vi "Configure Channel.vi"(4 "Vertical Offset (0.0 V)":dbl format="%.3p", 5 "Vertical Coupling (DC)":i32(slide)=1, 6 "Vertical Range (10.0 V)":dbl=10.0 format="%.2p", 7 "Channel Enabled (True)":bool=TRUE, 8 "error in (no error)":errorcluster {"code" format="%.0x"}, 9 "Probe Attenuation (1.0)":dbl=1.0 format="%.2f", 10 "Channel Name (\"CH1\")":string(combo)="CH1", 11 "VISA Resource Name":refnum<visa-resource-name>) -> (0 "error out":errorcluster {"code" format="%.0x"}, 3 "VISA Resource Name Out":refnum<visa-resource-name>)   [LabVIEW 2010, in "Tektronix TDS 3000 Series.lvlib"]
doc: "This VI configures the common properties of the oscilloscope's channel subsystem for a particular channel. These properties are the vertical range, vertical offset, coupling, probe attenuation, and channel enabled."
uses:
  <instrlib>/Tektronix TDS 3000 Series/Tektronix TDS 3000 Series.lvlib
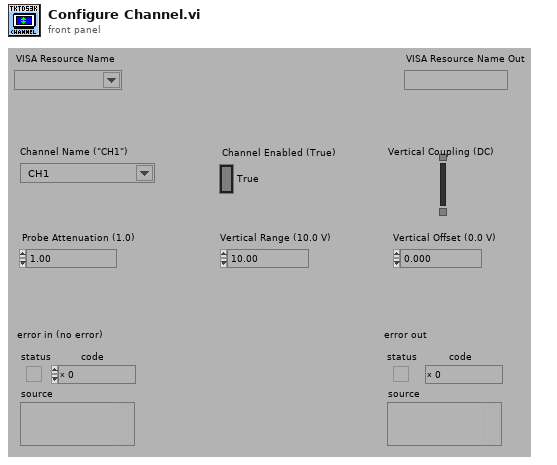
[diagram p1: front panel]
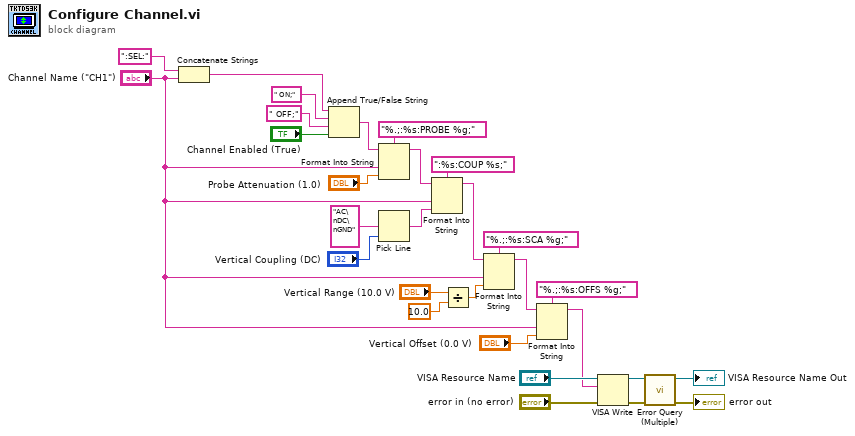
[diagram p0: block diagram]
diagram:
  n1 = Concatenate Strings(":SEL:" ("string"), "Channel Name (\"CH1\")") -> (w26:string)
  n2 = Append True/False String(1:"Channel Enabled (True)", 2:" OFF;" ("false string"), 3:" ON;" ("true string"), 4:w26) -> (0:w21:string)
  n3 = Format Into String(format string="%.;:%s:PROBE %g;", initial string=w21, "Channel Name (\"CH1\")", "Probe Attenuation (1.0)") -> (resulting string=w18:string)  [unwired: 1 in, 1 out]
  n4 = Pick Line(multi-line string="AC\nDC\nGND", line index="Vertical Coupling (DC)") -> (output string=w17:string)  [unwired: 1 in]
  n5 = Format Into String(format string=":%s:COUP %s;", initial string=w18, "Channel Name (\"CH1\")", w17) -> (resulting string=w14:string)  [unwired: 1 in, 1 out]
  n6 = Divide(x="Vertical Range (10.0 V)", y=10.0) -> (x/y=w8:dbl)
  n7 = Format Into String(format string="%.;:%s:SCA %g;", initial string=w14, "Channel Name (\"CH1\")", w8) -> (resulting string=w9:string)  [unwired: 1 in, 1 out]
  n8 = Format Into String(format string="%.;:%s:OFFS %g;", initial string=w9, "Channel Name (\"CH1\")", "Vertical Offset (0.0 V)") -> (resulting string=w10:string)  [unwired: 1 in, 1 out]
  n9 = VISA Write(VISA resource name="VISA Resource Name", write buffer=w10, error in (no error)="error in (no error)") -> (VISA resource name out=w4:refnum<visa-resource-name>, error out=w3:errorcluster)  [unwired: 1 out]
  n10 = call <instrlib>:"Error Query (Multiple).vi"("error in (no error)"=w3, "VISA Resource Name"=w4) -> ("error out"=→"error out":errorcluster, "VISA Resource Name Out"=→"VISA Resource Name Out":refnum<visa-resource-name>)  [unwired: 6 in, 2 out]
